vi "take_data (SubVI).vi"(2 "Synth_sync":bool, 3 "channel settings":T2={"samples per channel"=1000.0, "sampling rate"=1000.0, "data task"="", "Clock src"=""} {"sampling rate" format="%0.2f"}) -> (0 "data tasks":T1, 1 "Actual Sample Rate":dbl=10000.0 format="%0.2f")   [LabVIEW 2018]
uses:
  <vilib>/DAQmx/create/channels.llb/DAQmx Create Channel (AI-Voltage-Basic).vi
  <vilib>/DAQmx/configure/timing.llb/DAQmx Timing (Sample Clock).vi
  <vilib>/DAQmx/configure/trigger.llb/DAQmx Start Trigger (Digital Edge).vi
  <resource>/objmgr/daqmx.rc
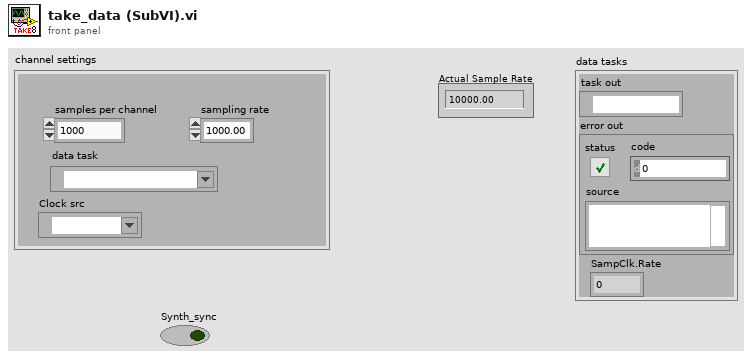
[diagram p1: front panel]
types:
  T1 = cluster{"task out":refnum<k21>, "error out":errorcluster, "SampClk.Rate":dbl}
  T2 = cluster{"samples per channel":dbl, "sampling rate":dbl, "data task":tag, "Clock src":tag}
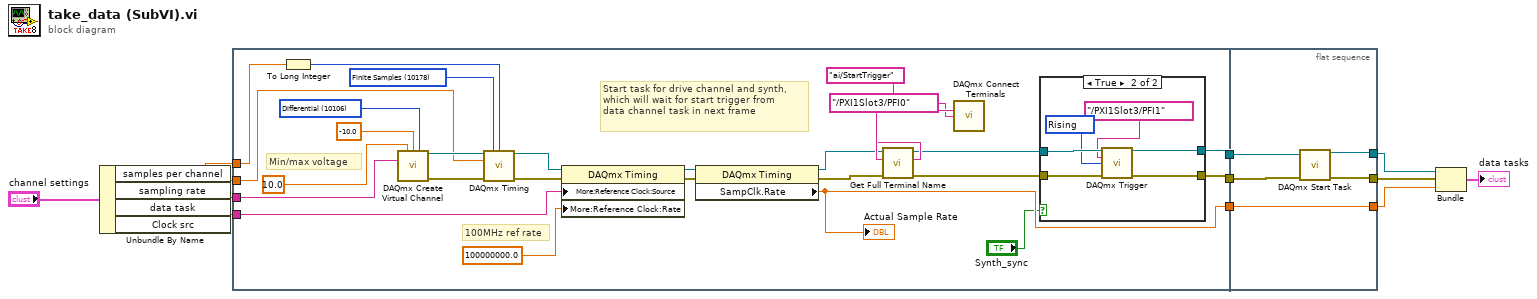
[diagram p0: block diagram]
diagram:
  n1 = Unbundle By Name("channel settings") -> ("samples per channel"=w7:dbl, "sampling rate"=w10:dbl, "data task"=w11:tag, "Clock src"=w6:tag)
  n2 = flat-sequence {
    tunnel: w11 -> [w31]
    tunnel: w10 -> [w26]
    tunnel: w7 -> [w23]
    tunnel: [w21] -> w4
    tunnel: [w20] -> w3
    tunnel: [w25] -> w2
    tunnel: w6 -> [w24]
    tunnel: [w52] -> w5
    tunnel: [w48] -> w8
    tunnel: [w49] -> w9
    tunnel: w2 -> [w52]
    tunnel: w3 -> [w50]
    tunnel: w4 -> [w51]
    frame #0 {
      w32 = 10106 items=["default"=-1, "RSE"=10083, "NRSE"=10078, "Differential"=10106, "Pseudodifferential"=12529] ("input terminal configuration")
      w28 = 10178 items=["Finite Samples"=10178, "Continuous Samples"=10123, "Hardware Timed Single Point"=12522] ("sample mode")
      # "Start task for drive channel and synth,\nwhich will wait for start trigger from \ndata channel task in next frame"
      # "100MHz ref rate"
      # "Min/max voltage"
      n3 = To Long Integer(number=w23) -> (32bit integer=w22:i32)
      n4 = call-poly <vilib>:"DAQmx Create Virtual Channel.vi"("maximum value"=10.0, "minimum value"=-10.0, "input terminal configuration"=w32, "physical channels"=w31) -> ("task out"=w33:refnum<k21>, "error out"=w34:errorcluster)  [unwired: 10 in]
      n5 = call-poly <vilib>:"DAQmx Timing.vi"("task/channels in"=w33, "sample mode"=w28, "samples per channel"=w22, "rate"=w26, "error in"=w34) -> ("task out"=w35:refnum<k21>, "error out"=w36:errorcluster)  [unwired: 9 in]
      n6 = property class="DAQmx Timing"(reference=w35, error in=w36, "More:Reference Clock:Source"=w24, "More:Reference Clock:Rate"=100000000.0 ("RefClk.Rate")) -> (reference out=w37:refnum<k21>, error out=w38:errorcluster)
      n7 = property class="DAQmx Timing"(reference=w37, error in=w38) -> (reference out=w16:refnum<k21>, error out=w15:errorcluster, "SampClk.Rate"=w25:dbl)
      "Actual Sample Rate" <- w25
      n8 = call "Get Full Terminal Name.vi"("error in (no error)"=w15, "Local Terminal Name"="ai/StartTrigger", "task/channels in"=w16) -> ("error out"=w13:errorcluster, "Terminal Name with Device Prefix"=w18:tag, "task out"=w14:refnum<k21>)  [unwired: 6 in]
      n9 = call <vilib>:"DAQmx Connect Terminals.vi"("source terminal"=w18, "destination terminal"=tag "/PXI1Slot3/PFI0" ("StartTrig.OutputTerm")) -> ()  [unwired: 13 in, 1 out]
      n10 = case shown="True" "Synth_sync" {
        tunnel: w14 -> [w40 w47]
        tunnel: [w40 w46] -> w21
        tunnel: w13 -> [w41 w43]
        tunnel: [w41 w42] -> w20
        frame False {
        }
        frame True {
          w44 = 10280 items=["Rising"=10280, "Falling"=10171] ("edge")
          n11 = call-poly <vilib>:"DAQmx Trigger.vi"("task/channels in"=w47, "source"=tag "/PXI1Slot3/PFI1", "edge"=w44, "error in"=w43) -> ("task out"=w46:refnum<k21>, "error out"=w42:errorcluster)  [unwired: 10 in]
        }
      }
    }
    frame #1 {
      n12 = call <vilib>:"DAQmx Start Task.vi"("task/channels in"=w51, "error in"=w50) -> ("task out"=w49:refnum<k21>, "error out"=w48:errorcluster)  [unwired: 12 in]
    }
  }
  n13 = Bundle("task out"=w9, "error out"=w8, "SampClk.Rate"=w5) -> (→"data tasks":T1)  [unwired: 1 in]
